vi "DarkSkyforLabVIEW.vi"   [LabVIEW 2017, in "Dark Sky Weather Data for LabVIEW.lvlib"]
uses:
  Dark Sky Weather Data for LabVIEW.lvlib
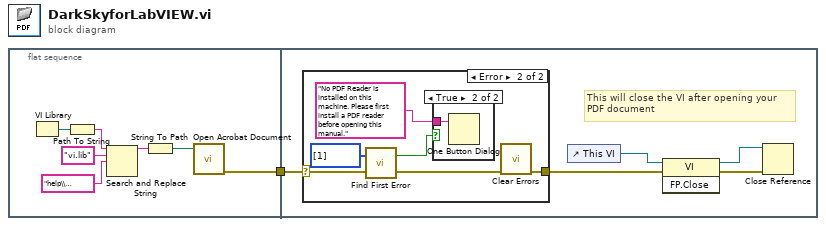
[diagram p0: block diagram]
diagram:
  n1 = flat-sequence {
    tunnel: [w8] -> w1
    tunnel: w1 -> [w10]
    frame #0 {
      n2 = VI Library() -> (path=w5:path)
      n3 = Path To String(path=w5) -> (string=w6:string)
      n4 = Search and Replace String(input string=w6, search string="vi.lib", replace string="help\\National Instruments\\Dark Sky Weather Data for LabVIEW\\Dark Sky for LabVIEW Help.pdf" ("replace string (\"\")")) -> (result string=w7:string)  [unwired: 5 in, 3 out]
      n5 = String To Path(string=w7) -> (path=w2:path)
      n6 = call <vilib>:"Open Acrobat Document.vi"("acrobat document"=w2) -> ("error out"=w8:errorcluster)  [unwired: 6 in]
    }
    frame #1 {
      # "This will close the VI after opening your\nPDF document"
      n7 = case shown="Error" w10 {
        selector: w10 -> [w14 w20]
        tunnel: [w14 w17] -> w9
        frame No Error {
        }
        frame Error {
          n8 = call <vilib>:"Find First Error.vi"("error in (no error)"=w20, "error codes"=i32[] [1]) -> ("error out"=w18:errorcluster, "error?"=w16:bool)  [unwired: 2 in]
          n9 = case shown="True" w16 {
            tunnel: "No PDF Reader is installed on this machine. Please first install a PDF reader before opening this manual." -> [_ w21]
            frame False {
            }
            frame True {
              n10 = One Button Dialog(message=w21) -> ()  [unwired: 1 in, 1 out]
            }
          }
          n11 = call <vilib>:"Clear Errors.vi"("error in (no error)"=w18) -> ("error out"=w17:errorcluster)  [unwired: 5 in, 1 out]
        }
      }
      n12 = control-ref of="This VI"() -> (w11:refnum<vi>)
      n13 = invoke class="VI" method="FP.Close"(reference=w11, error in=w9) -> (reference out=w13:refnum<vi>, error out=w12:errorcluster)  [unwired: 1 in, 1 out]
      n14 = Close Reference(reference=w13, error in (no error)=w12) -> ()  [unwired: 1 out]
    }
  }
